vi "Read Menue.vi"(8 "error in (no error)":errorcluster, 11 "MenueItem in":refnum<class "MenueItem.lvclass">) -> (0 "error out":errorcluster, 2 "Menue":refnum<k24>, 3 "MenueItem out":refnum<class "MenueItem.lvclass">)   [LabVIEW 2016, in "MenueItem.lvclass"]
uses:
  MenueItem.lvclass
  System.Windows.Forms
  MenueItem.lvclass/MenueItem.ctl
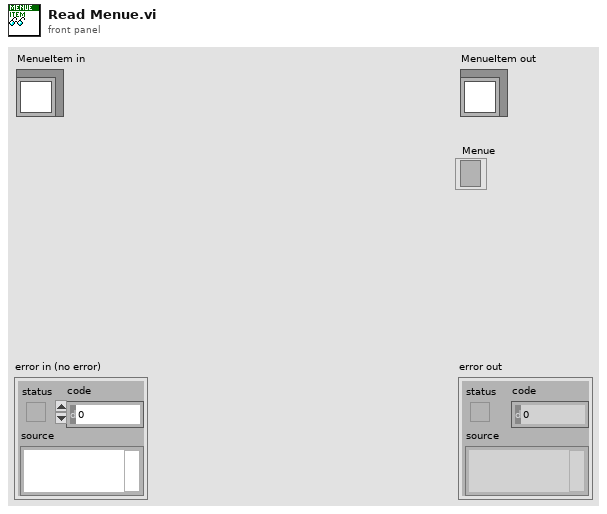
[diagram p1: front panel]
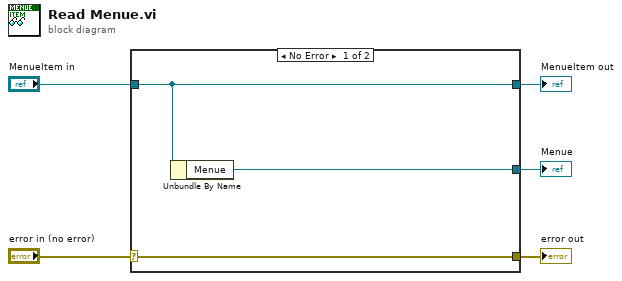
[diagram p0: block diagram]
diagram:
  n1 = case shown="No Error" "error in (no error)" {
    selector: "error in (no error)" -> [w8 w9]
    tunnel: [w8 w9] -> w4
    tunnel: [w7 w10] -> w2
    tunnel: "MenueItem in" -> [w7 w10]
    tunnel: [w6 _] -> w1
    frame No Error {
      n2 = Unbundle By Name(w7) -> ("Menue"=w6:refnum<k24>)
    }
    frame Error {
    }
  }
  "error out" <- w4
  "MenueItem out" <- w2
  "Menue" <- w1
